vi "写入项目.vi"(8 "error in (no error)":errorcluster caption="错误输入（无错误）", 10 "项目":u32(ring) items=["Amplitude", "Volts dc or update volts ac", "Volts ac dBm update", "Volts ac or volts dc with 0 Hz", "Volts ac in dBm", "Current dc or update current ac", "Current ac", "Update frequency", "Resistance", "Capacitance", "Temperature (Celsius)", "Temperature (Fahrenheit)", "Power dc or update power ac", "Power ac", "Dual volts dc or update dual ac", "Dual volts ac in volts", "Power ac in dBm update", "Power ac in dBm", "Dual volts ac in dBm update", "Dual volts ac in dBm"], 11 "多功能校准源接口输入":refnum<class "多功能校准源接口.lvclass">) -> (0 "error out":errorcluster caption="错误输出", 3 "多功能校准源接口输出":refnum<class "多功能校准源接口.lvclass">)   [LabVIEW 2020, in "多功能校准源接口.lvlib" / "多功能校准源接口.lvclass"]
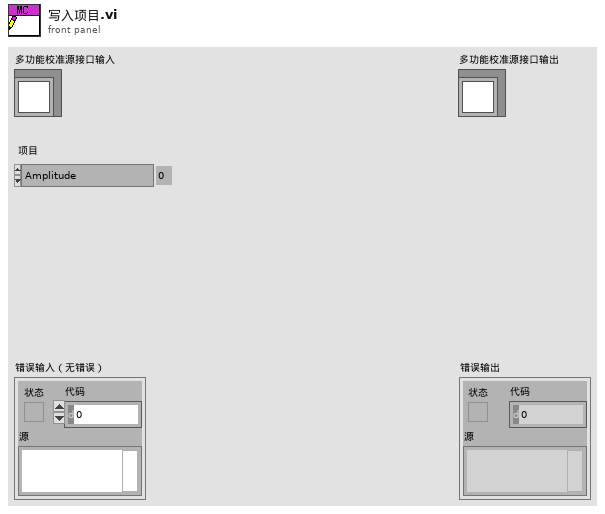
[diagram p1: front panel]
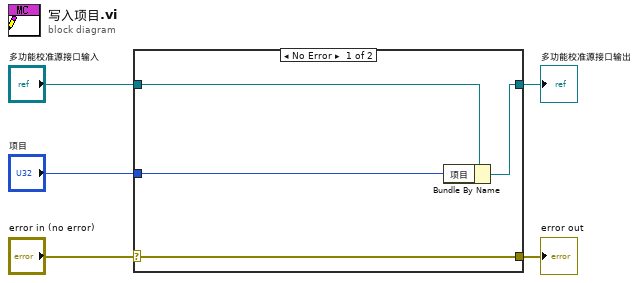
[diagram p0: block diagram]
diagram:
  n1 = case shown="No Error" "error in (no error)" {
    selector: "error in (no error)" -> [w9 w10]
    tunnel: [w9 w10] -> w4
    tunnel: [w7 w11] -> w2
    tunnel: "多功能校准源接口输入" -> [w8 w11]
    tunnel: "项目" -> [w6 _]
    frame No Error {
      n2 = Bundle By Name(cluster=w8, "项目"=w6) -> (w7:refnum<class "多功能校准源接口.lvclass">)
    }
    frame Error {
    }
  }
  "error out" <- w4
  "多功能校准源接口输出" <- w2
